vi "SendDIOProtocol.vi"(7 "Send":bool, 9 "Initiualize":bool, 10 "DIO old":T1={"type"="DIO", "device"="", "name"="", "data"={"<init"=FALSE, "<>value"=FALSE, "<pulse_length"=0, "<input"=FALSE}}, 11 "DIO new":T1={"type"="DIO", "device"="", "name"="", "data"={"<init"=FALSE, "<>value"=FALSE, "<pulse_length"=0, "<input"=FALSE}}) -> ()   [LabVIEW 2019]
uses:
  DIO proto.ctl
  DIO data proto.ctl
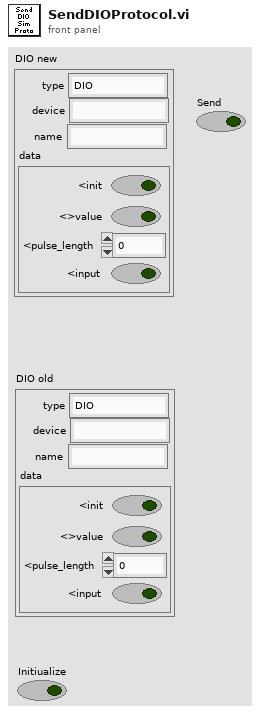
[diagram p1: front panel]
types:
  T1 = typedef "DIO proto.ctl" = cluster{"type":string, "device":string, "name":string, "data":T2}
  T2 = typedef "DIO data proto.ctl" = cluster{"<init":bool, "<>value":bool, "<pulse_length":i32, "<input":bool}
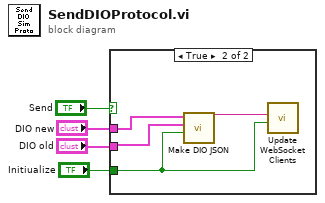
[diagram p0: block diagram]
diagram:
  n1 = case shown="True" "Send" {
    tunnel: "DIO new" -> [_ w8]
    tunnel: "DIO old" -> [_ w7]
    tunnel: "Initiualize" -> [_ w5]
    frame False {
    }
    frame True {
      n2 = call "Make DIO JSON.vi"("Force"=w5, "DIO prev"=w7, "DIO new"=w8) -> ("delta JSON"=w6:string)  [unwired: 8 in]
      n3 = call "Update WebSocket Clients.vi"("Initialize"=w5, "delta JSON"=w6) -> ()  [unwired: 10 in]
    }
  }
